vi "量測_VI_Pixel&mm.vi"(7 "Pixel轉mm":dbl, 8 "Distance右垂直(pixel)":dbl format="%.2f", 9 "Distances右水平(pixel)":dbl, 10 "Distance左垂直(pixel)":dbl format="%.2f", 11 "Distances左水平(pixel)":dbl) -> (0 "Distance右垂直(mm)":dbl, 1 "Distances右水平(mm)":dbl, 2 "Distance左垂直(mm)":dbl, 3 "Distances左水平(mm)":dbl)   [LabVIEW 2015]
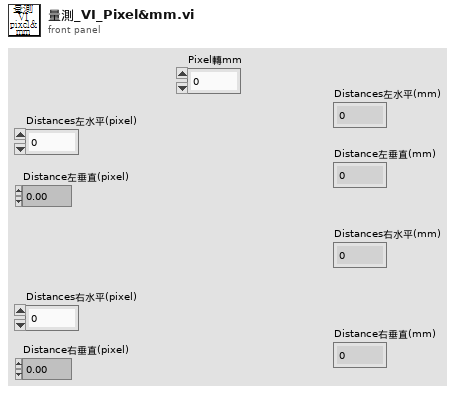
[diagram p1: front panel]
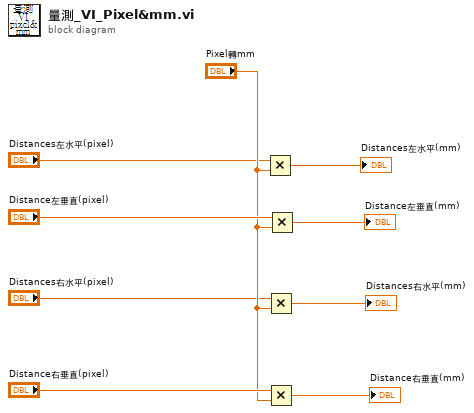
[diagram p0: block diagram]
diagram:
  n1 = Multiply(x="Distances左水平(pixel)", y="Pixel轉mm") -> (x*y=→"Distances左水平(mm)":dbl)
  n2 = Multiply(x="Distances右水平(pixel)", y="Pixel轉mm") -> (x*y=→"Distances右水平(mm)":dbl)
  n3 = Multiply(x="Distance右垂直(pixel)", y="Pixel轉mm") -> (x*y=→"Distance右垂直(mm)":dbl)
  n4 = Multiply(x="Distance左垂直(pixel)", y="Pixel轉mm") -> (x*y=→"Distance左垂直(mm)":dbl)
